vi "Configure UL-DL Periodicity.vi"(8 "error in (no error)":errorcluster, 9 "Periodicity (5 ms)":i32(ring)=7 items=["0.5 ms", "1 ms", "1.25 ms", "2 ms", "2.5 ms", "3 ms", "4 ms", "5 ms", "10 ms"], 10 "Instance (1)":T1=1, 11 "VISA resource name":refnum<visa-resource-name>) -> (0 "error out":errorcluster, 3 "VISA resource name out":refnum<visa-resource-name>)   [LabVIEW 2020, in "Rohde&Schwarz CMWXP NR FR1 Measurement.lvlib"]
doc: "Configures the periodicity of the TDD UL-DL pattern.\n\nAttribute:\nRSCMWXPNRFR1M_ATTR_UL_DL_PERIODICITY\n\nRemote-control command:\nCONFigure:NRSub:MEAS<i>:ULDL:PERiodicity"
uses:
  <instrlib>/Rohde&Schwarz CMWXP NR FR1 Measurement/Rohde&Schwarz CMWXP NR FR1 Measurement.lvlib
  <instrlib>/Rohde&Schwarz CMWXP NR FR1 Measurement/Private/_Instance.ctl
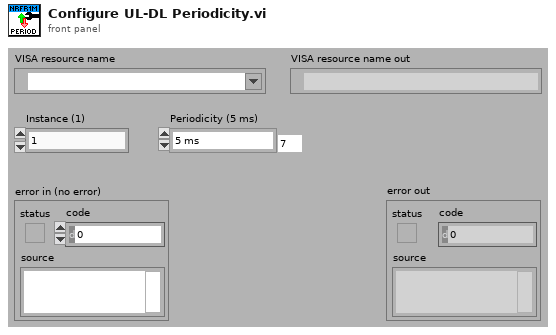
[diagram p1: front panel]
types:
  T1 = typedef "Rohde&Schwarz CMWXP NR FR1 Measurement.lvlib/_Instance.ctl" = i32
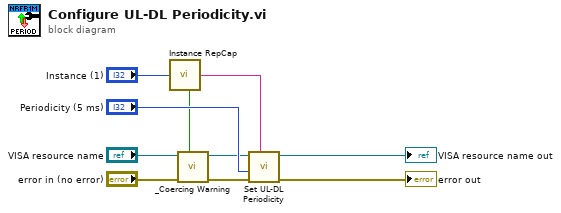
[diagram p0: block diagram]
diagram:
  n1 = call <instrlib>:"Instance RepCap.vi"("Instance In"="Instance (1)") -> ("In Range?"=w2:bool, "RepCap Identifier Out"=w6:string)  [unwired: 1 in]
  n2 = call <instrlib>:"_Coercing Warning.vi"("In Range?"=w2, "error in (no error)"="error in (no error)", "VISA resource name"="VISA resource name") -> ("error out"=w3:errorcluster, "VISA resource name out"=w1:refnum<visa-resource-name>)  [unwired: 7 in]
  n3 = call "Set UL-DL Periodicity"("Repeated Capabilities"=w6, "error in (no error)"=w3, "UL-DL Periodicity (0 - 0.5 ms)"="Periodicity (5 ms)", "instrument handle"=w1) -> ("error out"=→"error out":errorcluster, "instrument handle out"=→"VISA resource name out":refnum<visa-resource-name>)  [unwired: 6 in]
